vi "ScaleFirst.vi"(9 "Game Data":string, 10 "Start Point":T1(ring)) -> (2 "Scale First?":bool)   [LabVIEW 2017]
panel:
  # "True if scale first"
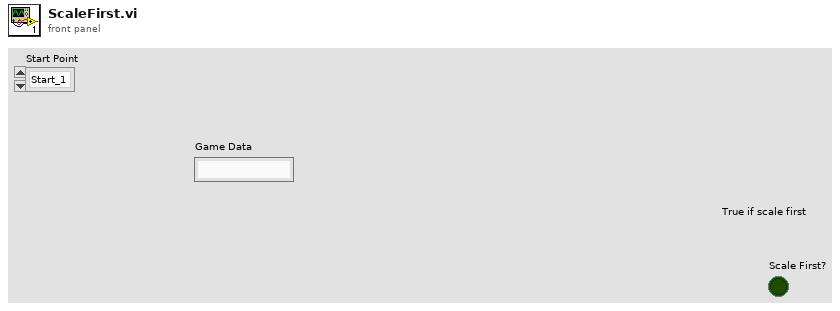
[diagram p1: front panel]
types:
  T1 = enum16{"Start_1", "Start_2", "Start_3", "Switch_L", "Switch_R", "Scale_L", "Scale_R", "Cube_1", "Cube_2", "Cube_3", "Cube_4", "Cube_5", "Cube_6", "CubeAcq_L", "CubeAcq_R", "Switch_Back_L", "Switch_Back_R"}
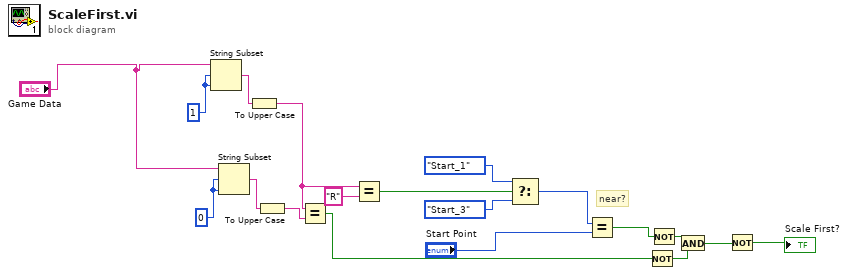
[diagram p0: block diagram]
diagram:
  w16 = 0 ("length (rest)")
  w18 = 1 ("length (rest)")
  # "near?"
  n1 = String Subset(string="Game Data", offset (0)=w18, length (rest)=w18) -> (substring=w19:string)
  n2 = String Subset(string="Game Data", offset (0)=w16, length (rest)=w16) -> (substring=w17:string)
  n3 = To Upper Case(1:w19) -> (0:w12:string)
  n4 = To Upper Case(1:w17) -> (0:w13:string)
  n5 = Equal?(x=w12, y=w13) -> (x = y?=w1:bool)
  n6 = Equal?(x=w12, y="R") -> (x = y?=w10:bool)
  n7 = Select(t=T1."Start_1" ("Start Point"), s=w10, f=T1."Start_3" ("Start Point")) -> (s? t:f=w7:T1)
  n8 = Equal?(x=w7, y="Start Point") -> (x = y?=w3:bool)
  n9 = Not(x=w1) -> (.not. x?=w2:bool)
  n10 = Not(x=w3) -> (.not. x?=w4:bool)
  n11 = And(x=w4, y=w2) -> (x .and. y?=w5:bool)
  n12 = Not(x=w5) -> (.not. x?=→"Scale First?":bool)
